vi "Periodic Tasks.vi"(8 "error in (no error)":errorcluster) -> ()   [LabVIEW 2015]
doc: "This VI runs in parallel to other tasks. It can contain as many user-defined periodic loops as you need. These can carry out PID or other sorts of timed response."
uses:
  <vilib>/Platform/TimedLoop/XDataNode/timing_clust.ctl
  <vilib>/Platform/TimedLoop/XDataNode/nitl_modes.ctl
  <vilib>/Platform/TimedLoop/XDataNode/wakeup.ctl
  Robot Global.vi
  <vilib>/platform/TimedLoop/XDataNode/XDataNode.xnode
  <vilib>/Platform/TimedLoop/XDataNode/XDNodeRunTimeDep.lvlib
panel:
  in  "Tare Currents?":bool
  out "all currents (A)":dbl[](array[numeric])
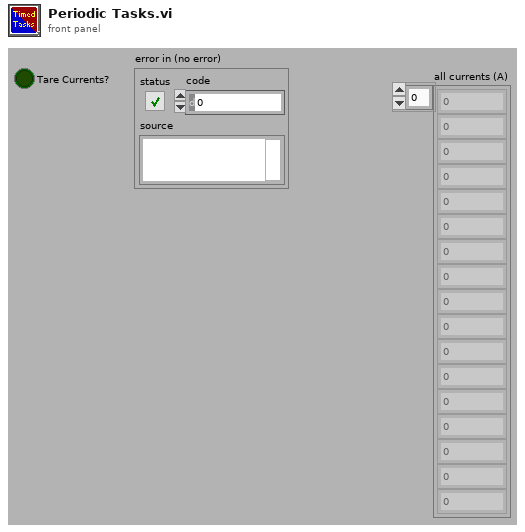
[diagram p1: front panel]
types:
  T1 = typedef "Robot Drive.ctl" = cluster{"RobotDriveDevRef":T2, "Joysticks":cluster{"JoystickDevRef":T10, "JoystickDevRef 2":T10}, "Sensor":T12, "Pneumatics":T31, "Defenses":cluster{"LeftArm MotorControlDeviceRef":T3, "RightArm MotorControlDeviceRef":T3}, "Hanging":cluster{"Left Erection MotorControlDeviceRef":T3, "Right Erection MotorControlDeviceRef":T3}, "Aquisition + Scoring":T35, "DigitalOutputDevRef":T39, "DigitalInputDevRef":T16}
  T2 = typedef "WPI_RobotDriveDevRef.ctl" = cluster{"DevStatus":errorcluster, "Motors[]":T3[], "Square Inputs":bool, "Max Output":dbl}
  T3 = typedef "WPI_MotorControlDeviceRef.ctl" = cluster{"DeviceStatus":errorcluster, "Type":T4, "PWM":cluster{"PWM Channel":T5, "DeadBand":T6}, "CAN":cluster{"Device Number":u8, "Control Mode":T7, "Semaphore":T8, "Max Vout":dbl, "TalonSRX Control Mode":T9}, "Invert":bool}
  T4 = typedef "WPI_MotorControlType.ctl" = enum16{"PWM", "CAN", "CANTalonSRX"}
  T5 = typedef "FPGA_DIOPWMChannel.ctl" = enum8{"PWM 0", "PWM 1", "PWM 2", "PWM 3", "PWM 4", "PWM 5", "PWM 6", "PWM 7", "PWM 8", "PWM 9", "PWM MXP 0", "PWM MXP 1", "PWM MXP 2", "PWM MXP 3", "PWM MXP 4", "PWM MXP 5", "PWM MXP 6", "PWM MXP 7", "PWM MXP 8", "PWM MXP 9", "Invalid"}
  T6 = typedef "WPI_PWMDeadband.ctl" = cluster{"Name":string, "maxPositivePwm":i32, "minPositivePwm":i32, "centerPwm":i32, "maxNegativePwm":i32, "minNegativePwm":i32, "angularRange":u16}
  T7 = typedef "WPI_CANJaguar_ControlMode.ctl" = enum8{"Percent VBus", "Current", "Speed", "Position", "Voltage"}
  T8 = typedef "Semaphore RefNum" = refnum<k1>
  T9 = typedef "WPI_CANTalonSRX_APIControlMode.ctl" = enum8{"Percent VBus", "Speed", "Position", "Slave", "Unchanged / Invalid", "Voltage Compensation", "Current", "Motion Profile"}
  T10 = typedef "WPI_JoystickDevRef.ctl" = cluster{"Device":T11}
  T11 = typedef "WPI_JoystickDeviceEnum.ctl" = enum16{"USB 0", "USB 1", "USB 2", "USB 3", "USB 4", "USB 5"}
  T12 = typedef "Sensors.ctl" = cluster{"GyroDevRef":T13, "Left Arm Limit DigitalInputDevRef":T16, "Right Arm Limit DigitalInputDevRef":T16, "Left Arm EncoderDevRef":T18, "Right Arm EncoderDevRef":T18, "Left Drive EncoderDevRef":T18, "Right Drive EncoderDevRef":T18, "BoB Photoeye DigitalInputDevRef":T16, "Range SonarMB1010AnalogDevRef":T22, "Shooter CounterDevRef":T24, "AccelerometerDevRef":T25, "Left Hanging Erecter EncoderDevRef":T18, "Right Hanging Erecter EncoderDevRef":T18, "TestDigitalInputDevRef":T16}
  T13 = typedef "WPI_GyroDevRef.ctl" = cluster{"DevStatus":errorcluster, "Analog Channel":T14, "Offset":dbl, "Gain (VoltsPerDegree/Second)":dbl, "Gyro Type":enum16{"Analog", "XRS450"}, "Handle":i32, "SPI Bus":T15, "Device Found":bool, "Sample Rate":dbl, "Calibrate On Open":bool}
  T14 = typedef "FPGA_AIChannel.ctl" = enum8{"AI 0", "AI 1", "AI 2", "AI 3", "AI MXP 0", "AI MXP 1", "AI MXP 2", "AI MXP 3", "Invalid"}
  T15 = typedef "spi_bus.ctl" = enum16{"SPI On-Board, CS0", "SPI On-Board, CS1", "SPI On-Board, CS2", "SPI On-Board, CS3", "SPI MXP", "Invalid"}
  T16 = typedef "WPI_DigitalInputDevRef.ctl" = cluster{"DevStatus":errorcluster, "DIO Channel":T17}
  T17 = typedef "FPGA_DIOChannel.ctl" = enum8{"DIO 0", "DIO 1", "DIO 2", "DIO 3", "DIO 4", "DIO 5", "DIO 6", "DIO 7", "DIO 8", "DIO 9", "DIO MXP 0", "DIO MXP 1", "DIO MXP 2", "DIO MXP 3", "DIO MXP 4", "DIO MXP 5", "DIO MXP 6", "DIO MXP 7", "DIO MXP 8", "DIO MXP 9", "DIO MXP 10", "DIO MXP 11", "DIO MXP 12", "DIO MXP 13", "DIO MXP 14", "DIO MXP 15", "Invalid"}
  T18 = typedef "WPI_EncoderDevRef.ctl" = cluster{"DevStatus":errorcluster, "EncoderIndex":T19, "CounterIndex":T20, "DistancePerCount":dbl, "Decoding Type":T21}
  T19 = typedef "FPGA_EncoderIdx.ctl" = enum8{"Enc 0", "Enc 1", "Enc 2", "Enc 3", "Enc 4", "Enc 5", "Enc 6", "Enc 7", "Invalid"}
  T20 = typedef "FPGA_CounterCtrSystemIndex.ctl" = enum8{"Ctr 0", "Ctr 1", "Ctr 2", "Ctr 3", "Ctr 4", "Ctr 5", "Ctr 6", "Ctr 7", "Invalid"}
  T21 = typedef "WPI_EncoderType.ctl" = enum16{"1x", "2x", "4x"}
  T22 = typedef "WPI_SonarMB1010AnalogDeviceRef.ctl" = cluster{"AIDeviceRef":T23, "Scaling factor (V/in)":dbl, "Average Bits":u8}
  T23 = typedef "WPI_AnalogChannelDevRef.ctl" = cluster{"DevStatus":errorcluster, "Analog Channel":T14}
  T24 = typedef "WPI_CounterDevRef.ctl" = cluster{"DevStatus":errorcluster, "CntIndex":T20}
  T25 = typedef "WPI_AccelerometerDevRef.ctl" = cluster{"DevStatus":errorcluster, "Scaling":T26, "Analog Channels":T27, "I2C Bus":T28, "SPI Bus":T15, "Accel Range":T29, "ADXL Axes":T30, "Handle":i32, "Device Address":u8, "Accel Type":enum16{"Analog", "ADXL345 I2C", "ADXL345 SPI", "Internal", "ADXL362 SPI"}}
  T26 = typedef "WPI_AccelerometerScaling.ctl" = cluster{"Gain (VoltsPerG)":dbl, "Center Voltage":dbl}
  T27 = typedef "WPI_AccelerometerAnalogChannels.ctl" = cluster{"X-Axis":T14, "Y-Axis":T14, "Z-Axis":T14}
  T28 = typedef "i2c_bus.ctl" = enum16{"I2C On-Board", "I2C MXP", "Invalid"}
  T29 = typedef "ADXL345 Range.ctl" = u8
  T30 = typedef "WPI_AccelerometerADXL345 Axes.ctl" = cluster{"X-Axis":bool, "Y-Axis":bool, "Z-Axis":bool}
  T31 = typedef "Pnematics.ctl" = cluster{"CompressorDevRef":T32, "High and Low Gear DoubleSolenoidDevRef":T33, "PTO SolenoidDevRef":T33, "Hang Pin SolenoidDevRef":T33}
  T32 = typedef "WPI_CompressorDevRef.ctl" = cluster{"DevStatus":errorcluster, "Pneumatics Control Module":u8}
  T33 = typedef "WPI_SolenoidDevRef.ctl" = cluster{"DevStatus":errorcluster, "Pneumatics Control Module":u8, "Forward Solenoid Channel":T34, "Reverse Solenoid Channel":T34}
  T34 = typedef "WPI_SolenoidChannel.ctl" = enum8{"Solenoid 0", "Solenoid 1", "Solenoid 2", "Solenoid 3", "Solenoid 4", "Solenoid 5", "Solenoid 6", "Solenoid 7", "Invalid"}
  T35 = typedef "Acquisition & Scoring.ctl" = cluster{"Outer Roller MotorControlDeviceRef":T3, "Inner Roller MotorControlDeviceRef":T3, "Scoring Top MotorControlDeviceRef":T3, "Scoring Bottom MotorControlDeviceRef":T3, "Flashlight RelayDevRef":T36}
  T36 = typedef "WPI_RelayDevRef.ctl" = cluster{"DevStatus":errorcluster, "Relay Channel":T37, "Relay Direction":T38}
  T37 = typedef "FPGA_DIORelayChannel.ctl" = enum8{"Relay 0", "Relay 1", "Relay 2", "Relay 3", "Invalid"}
  T38 = typedef "WPI_RelayDirection.ctl" = enum16{"Both directions", "Forward only", "Reverse only"}
  T39 = typedef "WPI_DigitalOutputDevRef.ctl" = cluster{"DIO Channel":T17, "DevStatus":errorcluster}
  T40 = cluster{"Left Erection MotorControlDeviceRef":T3, "Right Erection MotorControlDeviceRef":T3}
  T41 = typedef "XDNodeRunTimeDep.lvlib/timing_clust.ctl" = cluster{"Expected End [f-1]":u64, "Actual End [f-1]":u64, "Finished Late? [f-1]":bool, "Expected End [i-1]":u64, "Actual End [i-1]":u64, "Finished Late? [i-1]":bool, "Expected Start [i]":u64, "Actual Start [i]":u64, "Expected Start [f]":u64, "Actual Start [f]":u64, "Source Name":string, "Structure Name":string, "Period":i64, "Deadline":i64, "Offset":i64, "Start":i64, "Priority":i32, "Timeout":i32, "Mode":T42, "Wakeup Reason":T43, "Error":errorcluster, "Source Type":string, "Secondary Source Type":string, "Global End Time":u64, "Global Start Time":u64, "Frame Duration":u64, "Iteration Duration":u64, "Assigned CPU":i32, "I/O Scan Engine Mode":u32}
  T42 = typedef "XDNodeRunTimeDep.lvlib/nitl_modes.ctl" = enum32{"No Change", "Process missed periods, maintain original phase", "Discard missed periods, maintain original phase", "Process missed periods, ignore original phase", "Discard missed periods, ignore original phase"}
  T43 = typedef "XDNodeRunTimeDep.lvlib/wakeup.ctl" = enum32{"Normal", "Aborted", "Asynchronous wakeup", "Timing source error", "Timed loop error", "Timeout"}
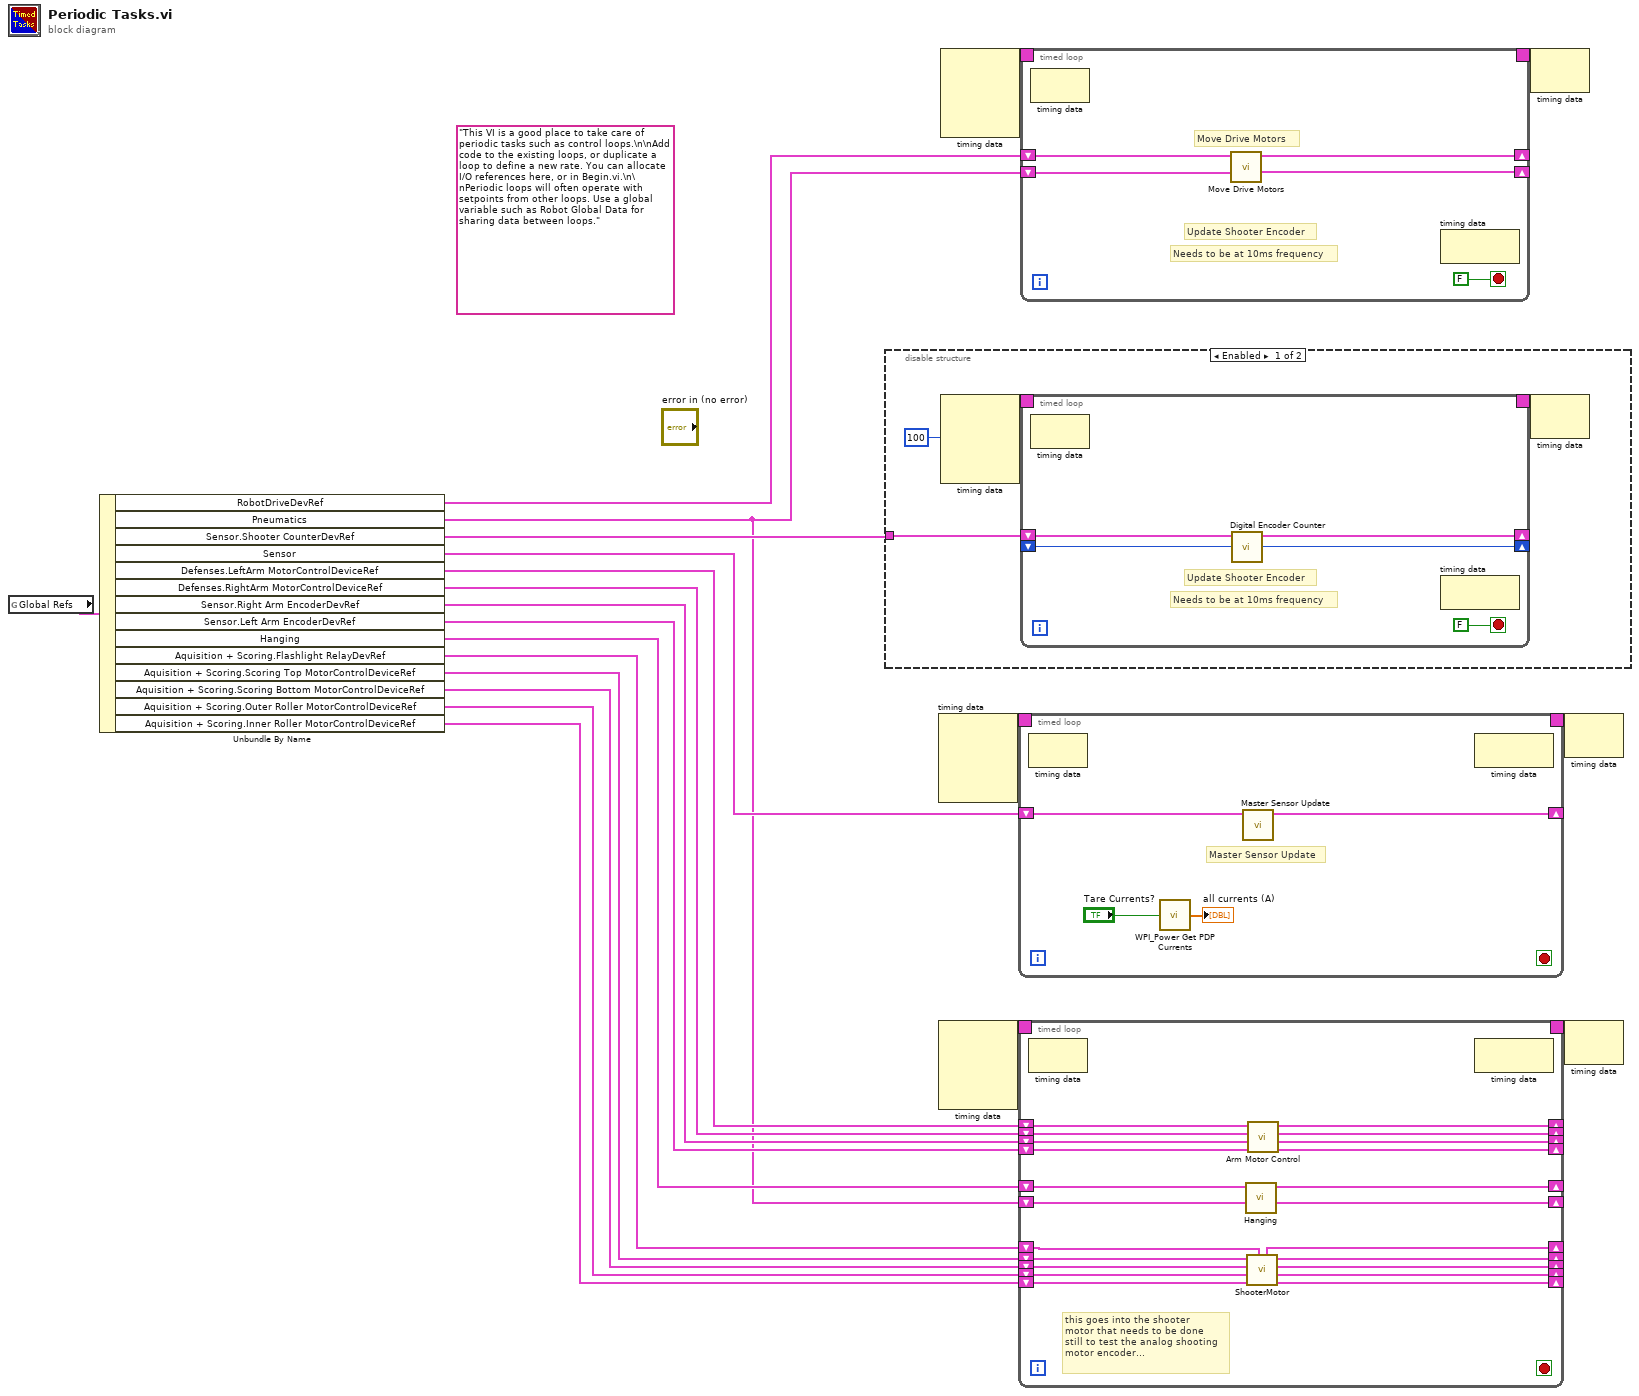
[diagram p0: block diagram]
diagram:
  (unwired) "This VI is a good place to take care of periodic tasks such as control loops.\n\nAdd code to the existing loops, or duplicate a loop to define a new rate. You can allocate I/O references here, or in Begin.vi.\n\nPeriodic loops will often operate with setpoints from other loops. Use a global variable such as Robot Global Data for sharing data between loops."
  n1 = global read "Robot Global.vi" "Global Refs"() -> (w21:T1)
  n2 = Unbundle By Name(w21) -> ("RobotDriveDevRef"=w7:T2, "Pneumatics"=w6:T31, "Sensor.Shooter CounterDevRef"=w18:T24, "Sensor"=w17:T12, "Defenses.LeftArm MotorControlDeviceRef"=w20:T3, "Defenses.RightArm MotorControlDeviceRef"=w19:T3, "Sensor.Right Arm EncoderDevRef"=w14:T18, "Sensor.Left Arm EncoderDevRef"=w13:T18, "Hanging"=w10:T40, "Aquisition + Scoring.Flashlight RelayDevRef"=w5:T36, "Aquisition + Scoring.Scoring Top MotorControlDeviceRef"=w16:T3, "Aquisition + Scoring.Scoring Bottom MotorControlDeviceRef"=w15:T3, "Aquisition + Scoring.Outer Roller MotorControlDeviceRef"=w12:T3, "Aquisition + Scoring.Inner Roller MotorControlDeviceRef"=w11:T3)
  n3 = disable-structure shown="Enabled" {
    disable-tunnel: w18 -> [w23 _]
    frame Enabled {
      n4 = node-c288(i64 100 ("Period")) -> (w25:T41)  [unwired: 3 in]
      n5 = timed-loop {
        timing: w25 -> [_]
        timing-out: [_] -> w24
        shift-right: [w27] -> _
        shift-left: w23 -> [w26]
        shift-right: [w29] -> _
        shift-left: _ -> [w28]
        stop <- FALSE stop-if-true
        # "Needs to be at 10ms frequency"
        # "Update Shooter Encoder"
        n6 = node-c288() -> ()  [unwired: 1 in, 1 out]
        n7 = call "Digital Encoder Counter.vi"("Previous Count"=w28, "Shooter CounterDevRef"=w26) -> ("Current Count"=w29:i32, "Shooter CounterDevRef 2"=w27:T24)  [unwired: 7 in, 1 out]
        n8 = node-c288() -> ()  [unwired: 1 in, 1 out]
      }
      n9 = node-c288(w24) -> ()  [unwired: 1 out]
    }
    frame Disabled {
    }
  }
  n10 = node-c288() -> (w4:T41)  [unwired: 4 in]
  n11 = node-c288() -> (w2:T41)  [unwired: 4 in]
  n12 = node-c288() -> (w9:T41)  [unwired: 4 in]
  n13 = timed-loop {
    timing: w4 -> [_]
    timing-out: [_] -> w3
    shift-right: [w39] -> _
    shift-left: w17 -> [w40]
    stop <- _ stop-if-true
    # "Master Sensor Update"
    n14 = node-c288() -> ()  [unwired: 1 in, 1 out]
    n15 = call <vilib>:"WPI_Power Get PDP Currents.vi"("Tare Currents?"="Tare Currents?") -> ("all currents (A)"=→"all currents (A)":dbl[])  [unwired: 12 in, 2 out]
    n16 = call "Master Sensor Update.vi"("Input"=w40) -> ("Output"=w39:T12)  [unwired: 10 in]
    n17 = node-c288() -> ()  [unwired: 1 in, 1 out]
  }
  n18 = timed-loop {
    timing: w2 -> [_]
    timing-out: [_] -> w1
    shift-right: [w62] -> _
    shift-left: w20 -> [w64]
    shift-right: [w61] -> _
    shift-left: w19 -> [w63]
    shift-right: [w58] -> _
    shift-left: w16 -> [w60]
    shift-right: [w57] -> _
    shift-left: w15 -> [w59]
    shift-right: [w54] -> _
    shift-left: w14 -> [w56]
    shift-right: [w53] -> _
    shift-left: w13 -> [w55]
    shift-right: [w51] -> _
    shift-left: w12 -> [w52]
    shift-right: [w49] -> _
    shift-left: w11 -> [w50]
    shift-right: [w47] -> _
    shift-left: w10 -> [w48]
    shift-right: [w45] -> _
    shift-left: w6 -> [w46]
    shift-right: [w43] -> _
    shift-left: w5 -> [w44]
    stop <- _ stop-if-true
    # "this goes into the shooter\nmotor that needs to be done\nstill to test the analog shooting\nmotor encoder..."
    n19 = node-c288() -> ()  [unwired: 1 in, 1 out]
    n20 = call "Hanging.vi"("Pneumatics In"=w46, "Hanging"=w48) -> ("Pneumatics Out"=w45:T31, "Hanging"=w47:T40)  [unwired: 8 in]
    n21 = call "ShooterMotor.vi"("RelayDevRef"=w44, "InnerRollerMtrRef"=w50, "OuterRollerMtrRef"=w52, "BottomShooterWheelMtrRef"=w59, "UpperShooterWheelMtrRef"=w60) -> ("InnerRollerMtrRef"=w49:T3, "OuterRollerMtrRef"=w51:T3, "BottomShooterWheelMtrRef"=w57:T3, "UpperShootWheelMtrRef"=w58:T3, "RelayDevRef 2"=w43:T36)  [unwired: 2 in]
    n22 = call "Arm Motor Control.vi"("Left Arm EncoderDevRef"=w55, "Right Arm EncoderDevRef"=w56, "Right Arm MotorControlDevRef"=w63, "Left Arm MotorControlDevRef"=w64) -> ("Left Arm EncoderDevRef"=w53:T18, "Right Arm EncoderDevRef"=w54:T18, "Right Arm MotorControlDevRef 2"=w61:T3, "Left Arm MotorControlDevRef 2"=w62:T3)  [unwired: 2 in]
    n23 = node-c288() -> ()  [unwired: 1 in, 1 out]
  }
  n24 = timed-loop {
    shift-right: [w69] -> _
    shift-left: w7 -> [w70]
    timing: w9 -> [_]
    timing-out: [_] -> w8
    shift-right: [w67] -> _
    shift-left: w6 -> [w68]
    stop <- FALSE stop-if-true
    # "Move Drive Motors"
    # "Needs to be at 10ms frequency"
    # "Update Shooter Encoder"
    n25 = node-c288() -> ()  [unwired: 1 in, 1 out]
    n26 = call "Move Drive Motors.vi"("Pneumatics In"=w68, "RobotDriveDevRef"=w70) -> ("Pneumatics Out"=w67:T31, "RobotDriveDevRef 2"=w69:T2)  [unwired: 8 in]
    n27 = node-c288() -> ()  [unwired: 1 in, 1 out]
  }
  n28 = node-c288(w8) -> ()  [unwired: 1 out]
  n29 = node-c288(w3) -> ()  [unwired: 1 out]
  n30 = node-c288(w1) -> ()  [unwired: 1 out]
